vi "language translator.vi"(6 "Language":T1, 11 "Language Data":T2) -> (1 "updated":bool, 3 "Language Data out":T2)   [LabVIEW 2015, in "AguaClara Library.lvlib"]
uses:
  AguaClara Library.lvlib
  Language.ctl
  Variable cluster.ctl
panel:
  in  "Load from VNG":bool
  in  "Table Control":string[][](table)
  in  "Cancel Button":bool caption="Cancelar"
  in  "OK Button":bool
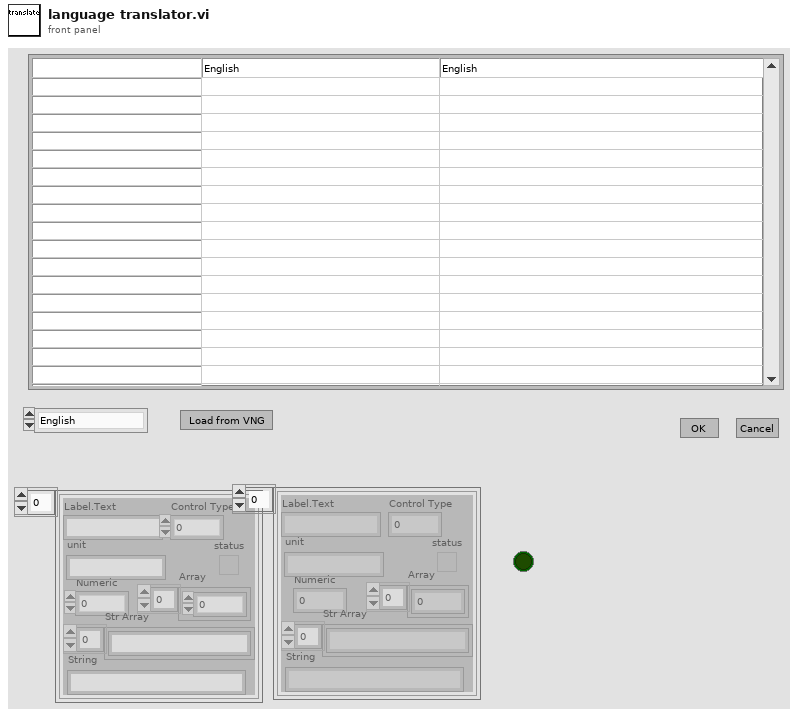
[diagram p1: front panel]
types:
  T1 = typedef "AguaClara Library.lvlib/Language.ctl" = enum16{"English", "Español", "French"}
  T2 = typedef "Variable cluster.ctl" = cluster{"Label.Text":string, "Control Type":u32, "Numeric":dbl, "Array":dbl[], "status":bool, "Str Array":string[], "String":string, "unit":string}[]
  T3 = cluster{"Label.Text":string, "Control Type":u32, "Numeric":dbl, "Array":dbl[], "status":bool, "Str Array":string[], "String":string, "unit":string}
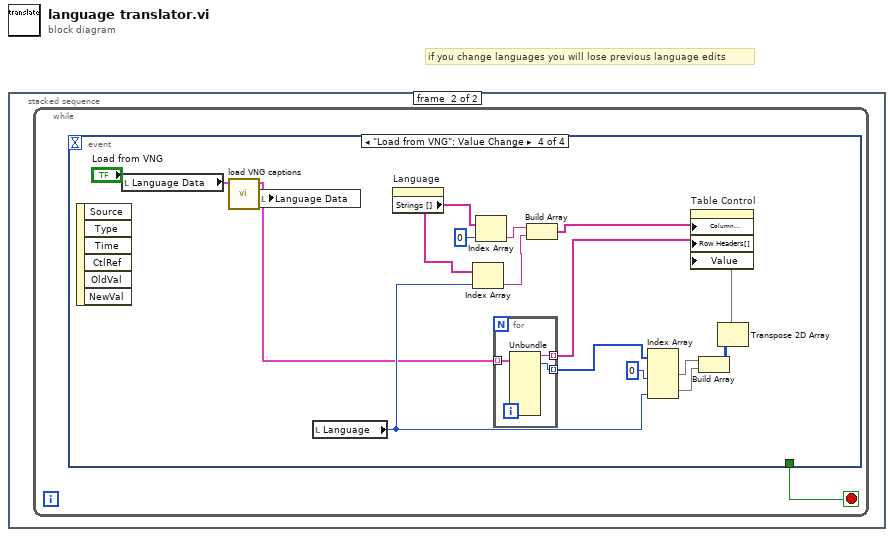
[diagram p0: block diagram]
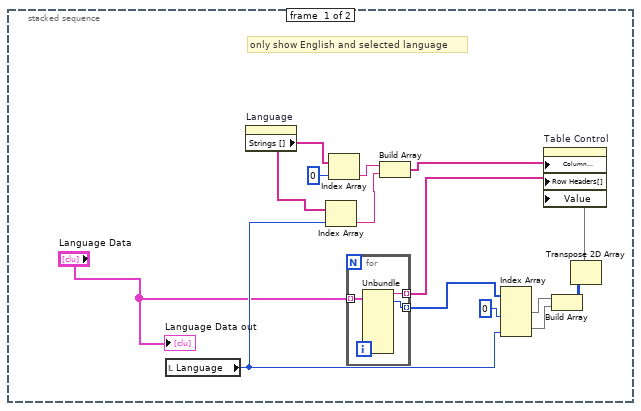
[diagram p2: hidden frame]
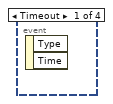
[diagram p3: hidden frame]
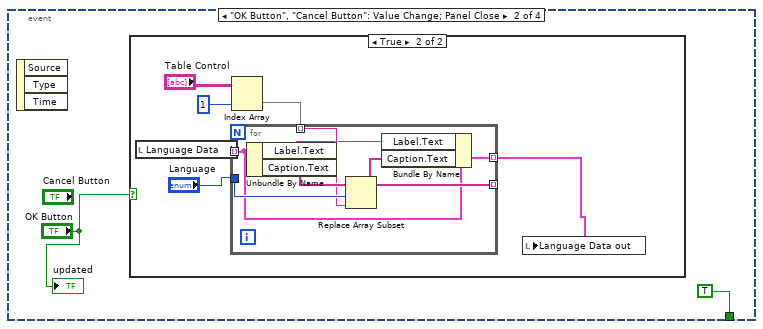
[diagram p4: hidden frame]
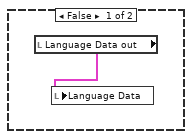
[diagram p5: hidden frame]
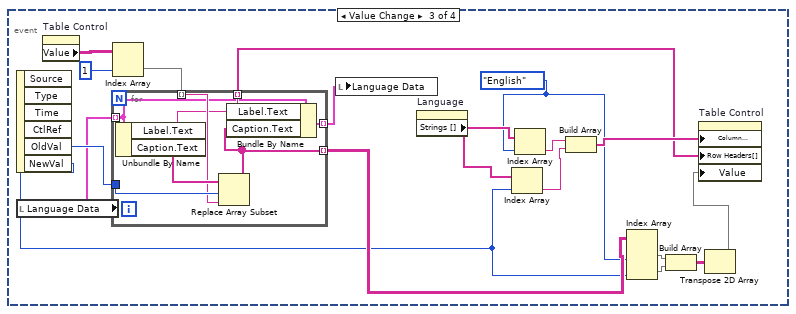
[diagram p6: hidden frame]
diagram:
  # "if you change languages you will lose previous language edits"
  n1 = stacked-sequence {
    frame #0 {
      # "only show English and selected language"
      n2 = local read "Language"() -> (w2:T1)
      n3 = property on="Language" class="Enum (strict)"() -> ("Strings []"=w14:string[])  [unwired: 2 in, 2 out]
      n4 = Index Array(array=w14, index=w2) -> (element=w11:string)
      n5 = Index Array(array=w14, index=0) -> (element=w12:string)
      n6 = for {
        tunnel: "Language Data" -> [w17] mode=indexing
        tunnel: [w16] -> w4 mode=indexing
        tunnel: [w15] -> w8 mode=indexing
        n7 = Unbundle(w17) -> ("Label.Text"=w16:string, "Control Type"=w15:u32)  [unwired: 6 out]
      }
      n8 = Build Array(w12, w11) -> (w5:string[])
      n9 = Index Array(array=w8, index (col) #1=0 ("index"), index (col) #2=w2) -> (element #1=w10:u32[], element #2=w7:u32[])  [unwired: 2 in]
      n10 = Build Array(w10, w7) -> (w9:u32[][])
      n11 = Transpose 2D Array(2D array=w9) -> (transposed array=w3:u32[][])
      n12 = property on="Table Control" class="Tbl (strict)"("Column Headers[]"=w5, "Row Headers[]"=w4, "Value"=w3) -> ()  [unwired: 2 in, 2 out]
      "Language Data out" <- "Language Data"
    }
    frame #1 {
      n13 = while {
        stop <- w18 stop-if-true
        n14 = event shown="[3] \"Load from VNG\": Value Change" {
          selector: _ -> [_ _ _ _]
          dyn-events: _ -> [_ _ _ _]
          timeout: _ -> [_ _ _ _]
          tunnel: [_ TRUE _ _] -> w18
          event Timeout {
            n15 = event-data() -> ()  [unwired: 1 in, 2 out]
          }
          event "OK Button", "Cancel Button": Value Change; Panel Close {
            n16 = event-data() -> ()  [unwired: 1 in, 3 out]
            n17 = case shown="True" "OK Button" {
              frame False {
                n18 = local read "Language Data out"() -> (w21:T2)
                n19 = local write "Language Data"(w21) -> ()
              }
              frame True {
                n20 = local read "Language Data"() -> (w26:T2)
                n21 = Index Array(array="Table Control", index (col)=1 ("index (row)")) -> (element=w27:string[])  [unwired: 1 in]
                n22 = for {
                  tunnel: w26 -> [w28] mode=indexing
                  tunnel: "Language" -> [w33]
                  tunnel: w27 -> [w32] mode=indexing
                  tunnel: [w31] -> w22 mode=indexing
                  tunnel: [w30] -> _ mode=indexing
                  n23 = Unbundle By Name(w28) -> ("Label.Text"=w29:string, "Caption.Text"=w34:string[])
                  n24 = Replace Array Subset(array=w34, new element=w32, index=w33) -> (w30:string[])
                  n25 = Bundle By Name(cluster=w28, "Label.Text"=w29, "Caption.Text"=w30) -> (w31:T3)
                }
                n26 = local write "Language Data out"(w22) -> ()
              }
            }
            "updated" <- "OK Button"
          }
          event Value Change {
            w35 = Language."English" ("Language")
            n27 = event-data() -> ("OldVal"=w43:T1, "NewVal"=w36:T1)  [unwired: 1 in, 4 out]
            n28 = local read "Language Data"() -> (w41:T2)
            n29 = property on="Table Control" class="Tbl (strict)"() -> ("Value"=w44:string[][])  [unwired: 2 in, 2 out]
            n30 = Index Array(array=w44, index (col)=1 ("index (row)")) -> (element=w42:string[])  [unwired: 1 in]
            n31 = for {
              tunnel: w41 -> [w53] mode=indexing
              tunnel: w43 -> [w58]
              tunnel: w42 -> [w57] mode=indexing
              tunnel: [w56] -> w40 mode=indexing
              tunnel: [w55] -> w39 mode=indexing
              tunnel: [w54] -> w38 mode=indexing
              n32 = Unbundle By Name(w53) -> ("Label.Text"=w54:string, "Caption.Text"=w59:string[])
              n33 = Replace Array Subset(array=w59, new element=w57, index=w58) -> (w55:string[])
              n34 = Bundle By Name(cluster=w53, "Label.Text"=w54, "Caption.Text"=w55) -> (w56:T3)
            }
            n35 = local write "Language Data"(w40) -> ()
            n36 = property on="Language" class="Enum (strict)"() -> ("Strings []"=w52:string[])  [unwired: 2 in, 2 out]
            n37 = Index Array(array=w52, index=w36) -> (element=w50:string)
            n38 = Index Array(array=w52, index=w35) -> (element=w51:string)
            n39 = Build Array(w51, w50) -> (w49:string[])
            n40 = Index Array(array=w39, index (col) #1=w35, index (col) #2=w36) -> (element #1=w48:string[], element #2=w46:string[])  [unwired: 2 in]
            n41 = Build Array(w48, w46) -> (w47:string[][])
            n42 = Transpose 2D Array(2D array=w47) -> (transposed array=w45:string[][])
            n43 = property on="Table Control" class="Tbl (strict)"("Column Headers[]"=w49, "Row Headers[]"=w38, "Value"=w45) -> ()  [unwired: 2 in, 2 out]
          }
          event "Load from VNG": Value Change {
            n44 = event-data() -> ()  [unwired: 1 in, 6 out]
            n45 = local read "Language Data"() -> (w74:T2)
            n46 = call "load VNG captions.vi"("Language Data In"=w74) -> ("Language Data Out"=w60:T2)  [unwired: 10 in]
            n47 = local write "Language Data"(w60) -> ()
            n48 = local read "Language"() -> (w61:T1)
            n49 = property on="Language" class="Enum (strict)"() -> ("Strings []"=w73:string[])  [unwired: 2 in, 2 out]
            n50 = Index Array(array=w73, index=w61) -> (element=w70:string)
            n51 = Index Array(array=w73, index=0) -> (element=w71:string)
            n52 = for {
              tunnel: w60 -> [w77] mode=indexing
              tunnel: [w76] -> w63 mode=indexing
              tunnel: [w75] -> w67 mode=indexing
              n53 = Unbundle(w77) -> ("Label.Text"=w76:string, "Control Type"=w75:u32)  [unwired: 6 out]
            }
            n54 = Build Array(w71, w70) -> (w64:string[])
            n55 = Index Array(array=w67, index (col) #1=0 ("index"), index (col) #2=w61) -> (element #1=w69:u32[], element #2=w66:u32[])  [unwired: 2 in]
            n56 = Build Array(w69, w66) -> (w68:u32[][])
            n57 = Transpose 2D Array(2D array=w68) -> (transposed array=w62:u32[][])
            n58 = property on="Table Control" class="Tbl (strict)"("Column Headers[]"=w64, "Row Headers[]"=w63, "Value"=w62) -> ()  [unwired: 2 in, 2 out]
          }
        }
      }
    }
  }
